vi "Batch_TriggerBuild.vi"(8 "error in (no error)":errorcluster, 11 "CommandLine":string[](array[string])) -> (0 "error out":errorcluster, 2 "test details":string, 3 "output to action":string)   [LabVIEW 2019]
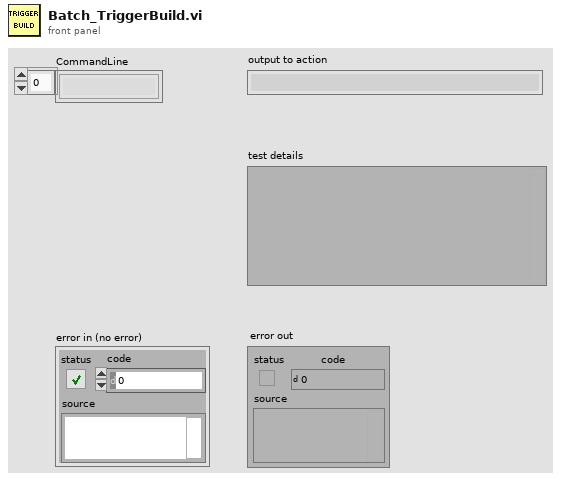
[diagram p1: front panel]
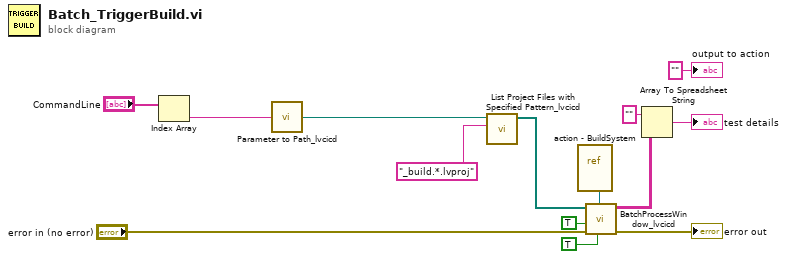
[diagram p0: block diagram]
diagram:
  n1 = Index Array(array="CommandLine") -> (element=w3:string)  [unwired: 1 in]
  n2 = call "Parameter to Path_lvcicd.vi"("String"=w3) -> ("Path"=w4:path)
  n3 = call "List Project Files with Specified Pattern_lvcicd.vi"("pattern"="_build.*.lvproj", "Path"=w4) -> ("All Files in Dir"=w8:path[])  [unwired: 7 in, 2 out]
  n4 = vi-ref "action - BuildSystem.vi"() -> (w10:refnum<vi>)
  n5 = call "BatchProcessWindow_lvcicd.vi"("FP(T)"=TRUE, "VI Refnum"=w10, "error in (no error)"="error in (no error)", "silence mode(F)"=TRUE, "paths"=w8) -> ("error out"=→"error out":errorcluster, "Array"=w13:string[][])  [unwired: 5 in]
  n6 = Array To Spreadsheet String(array=w13, 3:"" ("format string")) -> (spreadsheet string=→"test details":string)  [unwired: 1 in]
  "output to action" <- "" ("output to action")
